vi "Record Call.vi"(8 "error in (no error)":errorcluster, 10 "VI Call":refnum<class "VI Call.lvclass">, 11 "One Of In":refnum<class "One or More.lvclass">) -> (0 "error out":errorcluster, 3 "One Of Out":refnum<class "One or More.lvclass">)   [LabVIEW 2020, in "One or More.lvclass"]
uses:
  One or More.lvclass
  Core/VI Call/VI Call.lvclass
  One or More.lvclass/One or More.ctl
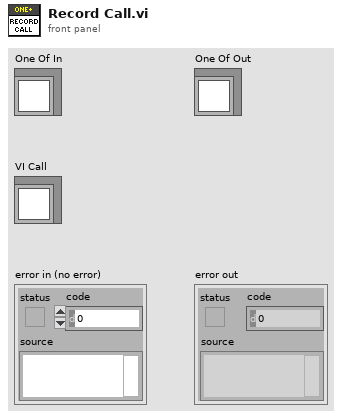
[diagram p1: front panel]
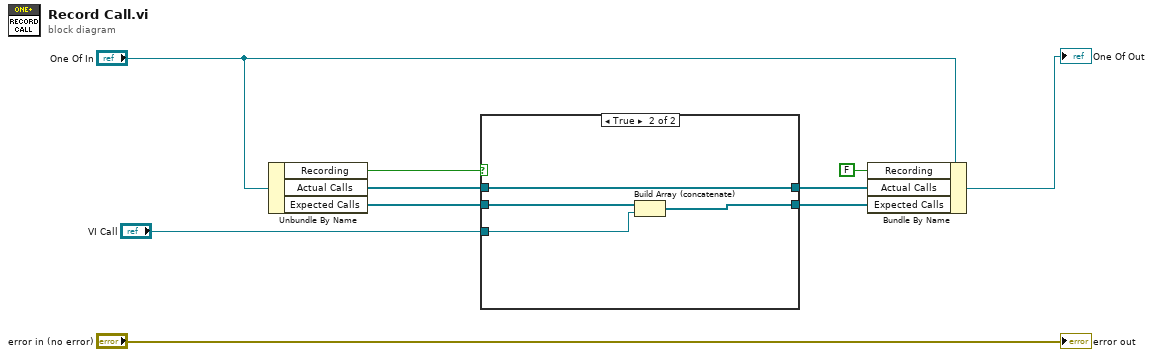
[diagram p0: block diagram]
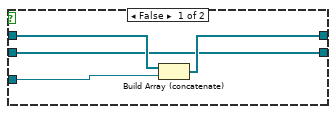
[diagram p2: hidden frame]
diagram:
  n1 = Unbundle By Name("One Of In") -> ("Recording"=w5:bool, "Actual Calls"=w9:refnum<class "VI Call.lvclass">[], "Expected Calls"=w3:refnum<class "VI Call.lvclass">[])
  n2 = case shown="True" w5 {
    tunnel: w9 -> [w14 w18]
    tunnel: [w13 w18] -> w8
    tunnel: "VI Call" -> [w11 w15]
    tunnel: w3 -> [w12 w17]
    tunnel: [w12 w16] -> w1
    frame False {
      n3 = Build Array (concatenate)(w14, w11) -> (w13:refnum<class "VI Call.lvclass">[])
    }
    frame True {
      n4 = Build Array (concatenate)(w17, w15) -> (w16:refnum<class "VI Call.lvclass">[])
    }
  }
  n5 = Bundle By Name(cluster="One Of In", "Recording"=FALSE, "Actual Calls"=w8, "Expected Calls"=w1) -> (→"One Of Out":refnum<class "One or More.lvclass">)
  "error out" <- "error in (no error)"
